vi "Demo.vi"() -> ()   [LabVIEW 2021, in "PS.lvlib"]
doc: "<b>Note:</b> This VI was modified by the <b>Validate DQMH Module</b> tool to turn off automatic error handling."
uses:
  PS.lvlib
  td_en_pstype.ctl
  f3b42825-7826-42e7-9565-ecda12019337.vi
panel:
  out "Output?":bool
  out "Curr Read":dbl
  out "Volt Read":dbl
  # "PS Demo"
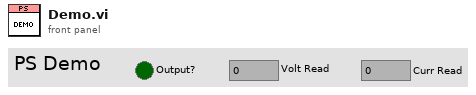
[diagram p1: front panel]
types:
  T1 = typedef "PS.lvlib/td_en_pstype.ctl" = enum16{"PS Simulated", "Keysight E3642A", "PS Test", "PS"}
  T2 = typedef "PS.lvlib/Get PS Data (Reply Payload)--cluster.ctl" = cluster{"Current":dbl, "Voltage":dbl, "Output?":bool, "error":errorcluster}
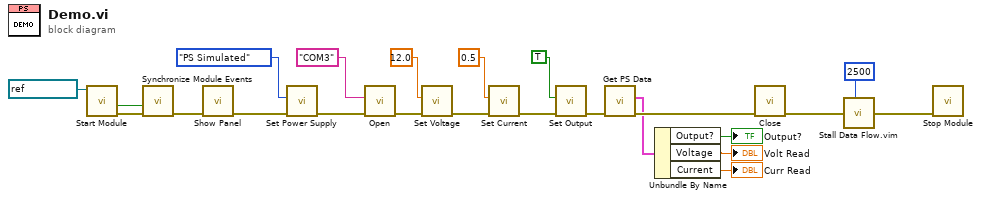
[diagram p0: block diagram]
diagram:
  n1 = call "Start Module.vi"("PS Type"=refnum<vi> refnum ("SubPanel")) -> ("error out"=w23:errorcluster, "Wait for Event Sync?"=w18:bool)  [unwired: 7 in, 2 out]
  n2 = call "Synchronize Module Events.vi"("error in (no error)"=w23, "Wait for Event Sync?"=w18) -> ("error out"=w22:errorcluster)  [unwired: 9 in]
  n3 = call "Show Panel.vi"("error in (no error)"=w22) -> ("error out"=w5:errorcluster)  [unwired: 10 in]
  n4 = call "Set Power Supply.vi"("error in (no error)"=w5, "Power Supply class"=td_en_pstype."PS Simulated") -> ("error out"=w11:errorcluster)  [unwired: 9 in]
  n5 = call "Open.vi"("error in"=w11, "Resource"="COM3") -> ("error out"=w21:errorcluster)  [unwired: 8 in, 1 out]
  n6 = call "Set Voltage.vi"("error in"=w21, "Voltage"=12.0) -> ("error out"=w20:errorcluster)  [unwired: 9 in]
  n7 = call "Set Current.vi"("error in"=w20, "Curr"=0.5) -> ("error out"=w19:errorcluster)  [unwired: 9 in]
  n8 = call "Set Output.vi"("error in"=w19, "Output?"=TRUE) -> ("error out"=w14:errorcluster)  [unwired: 9 in]
  n9 = call "Get PS Data.vi"("error in"=w14) -> ("error out"=w13:errorcluster, "PS Data"=w12:T2)  [unwired: 8 in, 1 out]
  n10 = Unbundle By Name(w12) -> ("Output?"=→"Output?":bool, "Voltage"=→"Volt Read":dbl, "Current"=→"Curr Read":dbl)
  n11 = call "Close.vi"("error in"=w13) -> ("error out"=w3:errorcluster)  [unwired: 9 in, 1 out]
  n12 = call "Stall Data Flow.vim"("value in"=w3, "milliseconds to wait"=u32 2500) -> ("value out"=w2:errorcluster)  [unwired: 1 out]
  n13 = call "Stop Module.vi"("error in (no error)"=w2) -> ()  [unwired: 10 in, 1 out]
